vi "Create Class from Template.vi"(8 "Error In":errorcluster, 9 "Target Name":string, 10 "Target Path":path, 11 "Template Class":path) -> (0 "Error Out":errorcluster, 3 "New Lib Path":path)   [LabVIEW 2011, in "Generator.lvlib"]
doc: "This VI saves a copy of an existing Class to the <B>Target Location</B> with <B>Target Name</B>."
uses:
  Generator.lvlib
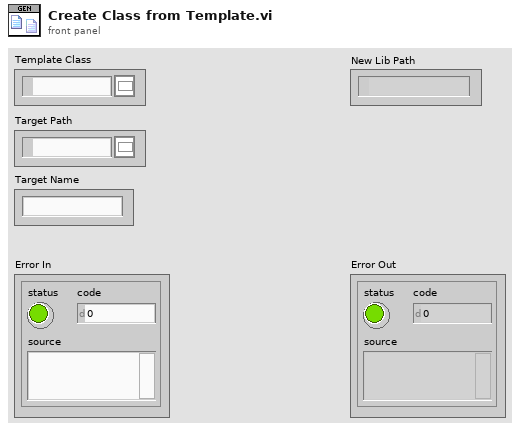
[diagram p1: front panel]
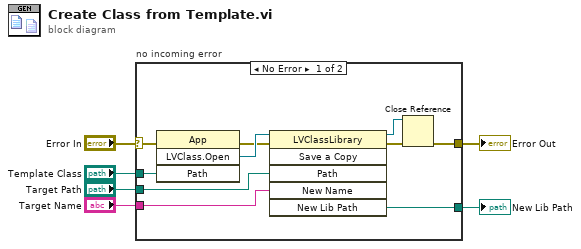
[diagram p0: block diagram]
diagram:
  n1 = case "no incoming error" shown="No Error" "Error In" {
    selector: "Error In" -> [w16 w17]
    tunnel: [w8 w17] -> w5
    tunnel: "Template Class" -> [w15 _]
    tunnel: "Target Path" -> [w12 _]
    tunnel: "Target Name" -> [w11 _]
    tunnel: [w7 _] -> w1
    frame No Error {
      n2 = invoke class="App" method="LVClass.Open"(error in=w16, "Path"=w15) -> (error out=w13:errorcluster, "LVClass.Open"=w14:refnum<vi>)  [unwired: 2 in, 2 out]
      n3 = invoke class="LVClassLibrary" method="Save a Copy"(reference=w14, error in=w13, "Path"=w12, "New Name"=w11) -> (reference out=w9:refnum<vi>, error out=w10:errorcluster, "New Lib Path"=w7:path)  [unwired: 2 in, 3 out]
      n4 = Close Reference(reference=w9, error in (no error)=w10) -> (error out=w8:errorcluster)
    }
    frame Error {
    }
  }
  "Error Out" <- w5
  "New Lib Path" <- w1
